vi "TSCAN_SignalTable.vi"(10 "Buffer":T1(array[cluster]), 11 "MCListbox reference handle":refnum<vi>) -> ()   [LabVIEW 2014]
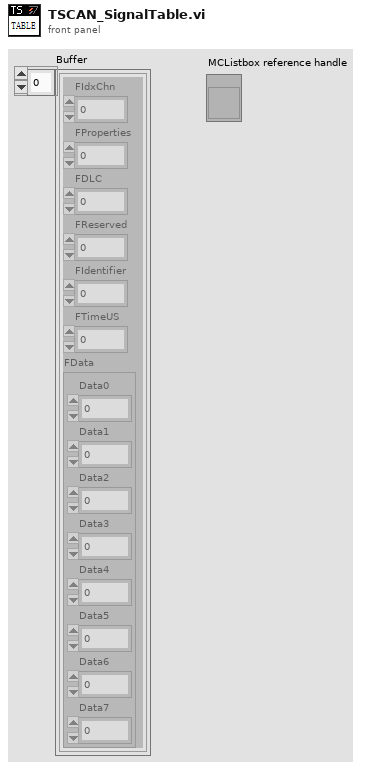
[diagram p1: front panel]
types:
  T1 = cluster{"FIdxChn":u8, "FProperties":u8, "FDLC":u8, "FReserved":u8, "FIdentifier":i32, "FTimeUS":u64, "FData":cluster{"Data0":u8, "Data1":u8, "Data2":u8, "Data3":u8, "Data4":u8, "Data5":u8, "Data6":u8, "Data7":u8}}[]
  T2 = cluster{"Data0":u8, "Data1":u8, "Data2":u8, "Data3":u8, "Data4":u8, "Data5":u8, "Data6":u8, "Data7":u8}
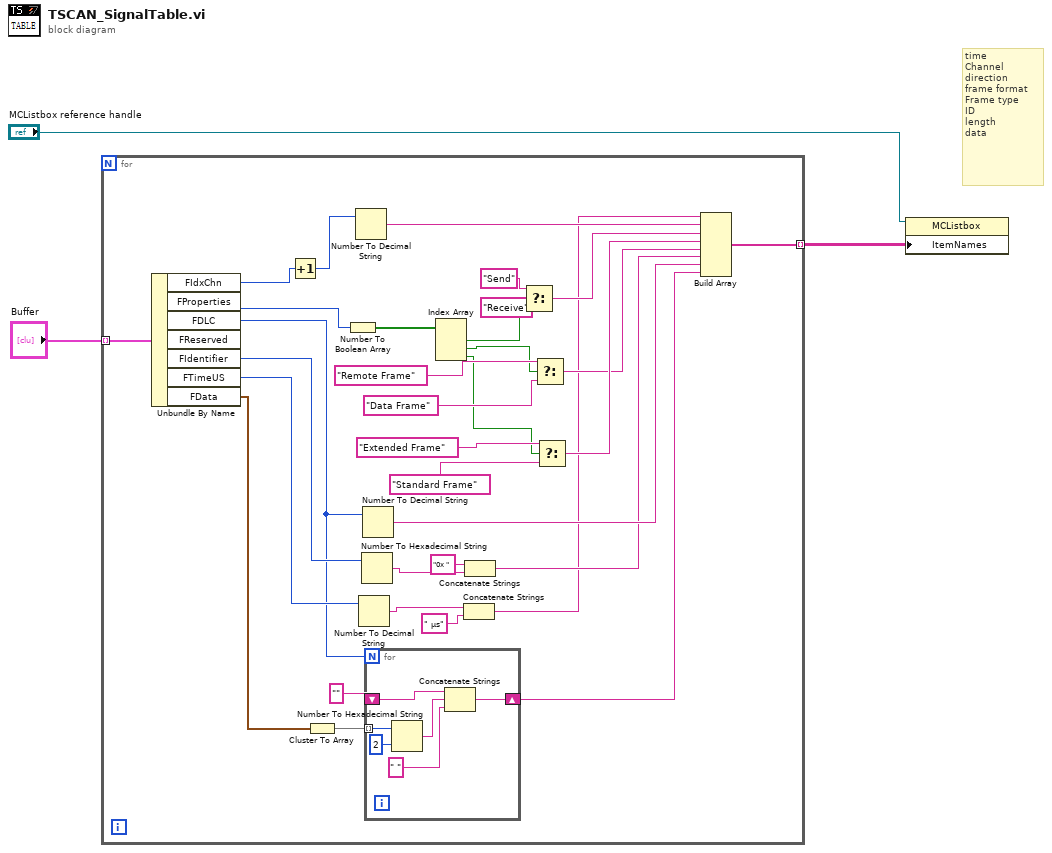
[diagram p0: block diagram]
diagram:
  # "time\nChannel\ndirection\nframe format\nFrame type\nID\nlength\ndata"
  n1 = for {
    tunnel: "Buffer" -> [w36] mode=indexing
    tunnel: [w12] -> w3 mode=indexing
    n2 = Unbundle By Name(w36) -> ("FIdxChn"=w11:u8, "FProperties"=w35:u8, "FDLC"=w20:u8, "FIdentifier"=w24:i32, "FTimeUS"=w23:u64, "FData"=w21:T2)  [unwired: 1 out]
    n3 = Increment(x=w11) -> (x+1=w10:u8)
    n4 = Cluster To Array(cluster=w21) -> (array=w19:u8[])
    n5 = Number To Boolean Array(number=w35) -> (Boolean array=w34:bool[])
    n6 = Number To Decimal String(number=w10) -> (decimal integer string=w18:string)  [unwired: 1 in]
    n7 = Number To Decimal String(number=w23) -> (decimal integer string=w5:string)  [unwired: 1 in]
    n8 = Number To Hexadecimal String(2:w24) -> (0:w8:string)  [unwired: 1 in]
    n9 = Number To Decimal String(number=w20) -> (decimal integer string=w14:string)  [unwired: 1 in]
    n10 = for {
      N: w20 -> [_]
      tunnel: w19 -> [w39] mode=indexing
      shift-right: [w41] -> w13
      shift-left: "" -> [w42]
      n11 = Number To Hexadecimal String(1:i16 2 ("width (-)"), 2:w39) -> (0:w38:string)
      n12 = Concatenate Strings(w42, w38, " " ("string")) -> (w41:string)
    }
    n13 = Index Array(array=w34) -> (element #1=w33:bool, element #2=w28:bool, element #3=w25:bool)  [unwired: 3 in]
    n14 = Concatenate Strings(w5, " μs" ("字符串")) -> (w6:string)
    n15 = Concatenate Strings("0x " ("字符串"), w8) -> (w9:string)
    n16 = Select(t="Send", s=w33, f="Receive") -> (s? t:f=w17:string)
    n17 = Select(t="Remote Frame", s=w28, f="Data Frame") -> (s? t:f=w15:string)
    n18 = Select(t="Extended Frame", s=w25, f="Standard Frame") -> (s? t:f=w16:string)
    n19 = Build Array(w6, w18, w17, w16, w15, w9, w14, w13) -> (w12:string[])
  }
  n20 = property class="MCListbox"(reference="MCListbox reference handle", "ItemNames"=w3) -> ()  [unwired: 1 in, 2 out]
